vi "H.vi"(3 "t":ext, 4 "n^2":ext, 5 "Promien krzywizny południka [v]":ext, 6 "fi[rad]":ext) -> (0 "H":ext)   [LabVIEW 2012, in "Biblioteka moduł map v3.lvlib" / "Konwersja wsp.lvlib" / "UTM.lvlib" / "Konwersja na UTM.lvlib"]
doc: "Współczynnik wzoru na konwersję na UTM."
uses:
  Konwersja na UTM.lvlib
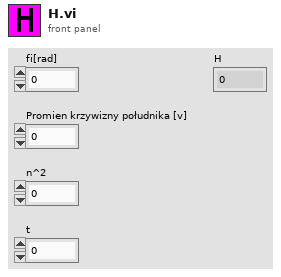
[diagram p1: front panel]
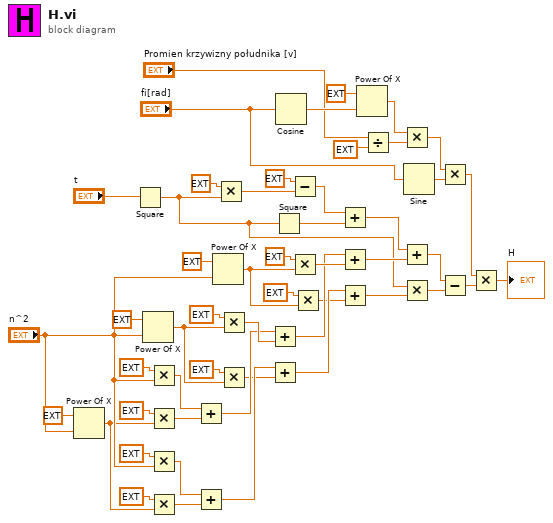
[diagram p0: block diagram]
diagram:
  n1 = Power Of X(1:"n^2", 2:ext 2.0 ("y")) -> (0:w4:ext)
  n2 = Square(x="t") -> (x^2=w16:ext)
  n3 = Power Of X(1:"n^2", 2:ext 3.0 ("y")) -> (0:w3:ext)
  n4 = Multiply(x=ext 270.0, y="n^2") -> (x*y=w30:ext)
  n5 = Multiply(x=ext 445.0, y=w4) -> (x*y=w28:ext)
  n6 = Multiply(x=ext 330.0, y="n^2") -> (x*y=w7:ext)
  n7 = Multiply(x=ext 680.0, y=w4) -> (x*y=w9:ext)
  n8 = Add(x=w30, y=w28) -> (x+y=w25:ext)
  n9 = Add(x=w7, y=w9) -> (x+y=w12:ext)
  n10 = Power Of X(1:"n^2", 2:ext 4.0 ("y")) -> (0:w2:ext)
  n11 = Multiply(x=ext 58.0, y=w16) -> (x*y=w38:ext)
  n12 = Multiply(x=ext 324.0, y=w3) -> (x*y=w27:ext)
  n13 = Multiply(x=ext 600.0, y=w3) -> (x*y=w10:ext)
  n14 = Add(x=w25, y=w27) -> (x+y=w22:ext)
  n15 = Add(x=w12, y=w10) -> (x+y=w15:ext)
  n16 = Square(x=w16) -> (x^2=w36:ext)
  n17 = Cosine(x="fi[rad]") -> (cos(x)=w47:ext)
  n18 = Subtract(x=ext 61.0, y=w38) -> (x-y=w35:ext)
  n19 = Multiply(x=ext 88.0, y=w2) -> (x*y=w23:ext)
  n20 = Multiply(x=ext 192.0, y=w2) -> (x*y=w14:ext)
  n21 = Add(x=w35, y=w36) -> (x+y=w21:ext)
  n22 = Add(x=w22, y=w23) -> (x+y=w20:ext)
  n23 = Add(x=w15, y=w14) -> (x+y=w1:ext)
  n24 = Power Of X(1:w47, 2:ext 5.0 ("y")) -> (0:w49:ext)
  n25 = Divide(x="Promien krzywizny południka [v]", y=ext 720.0) -> (x/y=w50:ext)
  n26 = Multiply(x=w49, y=w50) -> (x*y=w51:ext)
  n27 = Add(x=w21, y=w20) -> (x+y=w19:ext)
  n28 = Multiply(x=w16, y=w1) -> (x*y=w17:ext)
  n29 = Sine(x="fi[rad]") -> (sin(x)=w43:ext)
  n30 = Multiply(x=w51, y=w43) -> (x*y=w42:ext)
  n31 = Subtract(x=w19, y=w17) -> (x-y=w18:ext)
  n32 = Multiply(x=w42, y=w18) -> (x*y=→"H":ext)
